vi "bar_code_reader.vi"() -> ()   [LabVIEW 2011]
doc: "This example shows how to use the IMAQ Read Barcode VI to read standard 1D barcodes.\n\nThe images are loaded with the Vision Acquisition Software Express VI."
uses:
  <vilib>/userDefined/High Color/IMAQdx.ctl
  <vilib>/vision/driver/IMAQdx.llb/IMAQdx Acquisition Mode.ctl
  <vilib>/vision/driver/IMAQdx.llb/IMAQdx Buffer Number Mode.ctl
  <vilib>/vision/NI_Vision_Development_Module.lvlib
  <vilib>/vision/driver/NI_Vision_Acquisition_Software.lvlib
panel:
  out "Code 4":string
  in  "Barcode Type":u32(ring)=6 items=["Reserved", "Codabar", "Code 39", "Code 93", "Code 128", "EAN 8", "EAN 13", "Interleaved 2 of 5", "MSI", "UPCA"]
  in  "Boolean 2":bool
  out "Code 3":string
  in  "Boolean":bool
  out "Code 2":string
  out "Acquisition Rate (frames/s)":dbl(knob) scale=0.0..110.0
  in  "stop 2":bool
  in  "Camera Name":T1
  out "Image":T2(plugin-control) caption="Draw a Rectangular Region of Interest on the BarCode"
  in  "Delay (ms)":i32(slide)=1446 max=3000 scale=0.0..100000.0
  # "This example requires Vision Acquisition Express VI to be installed"
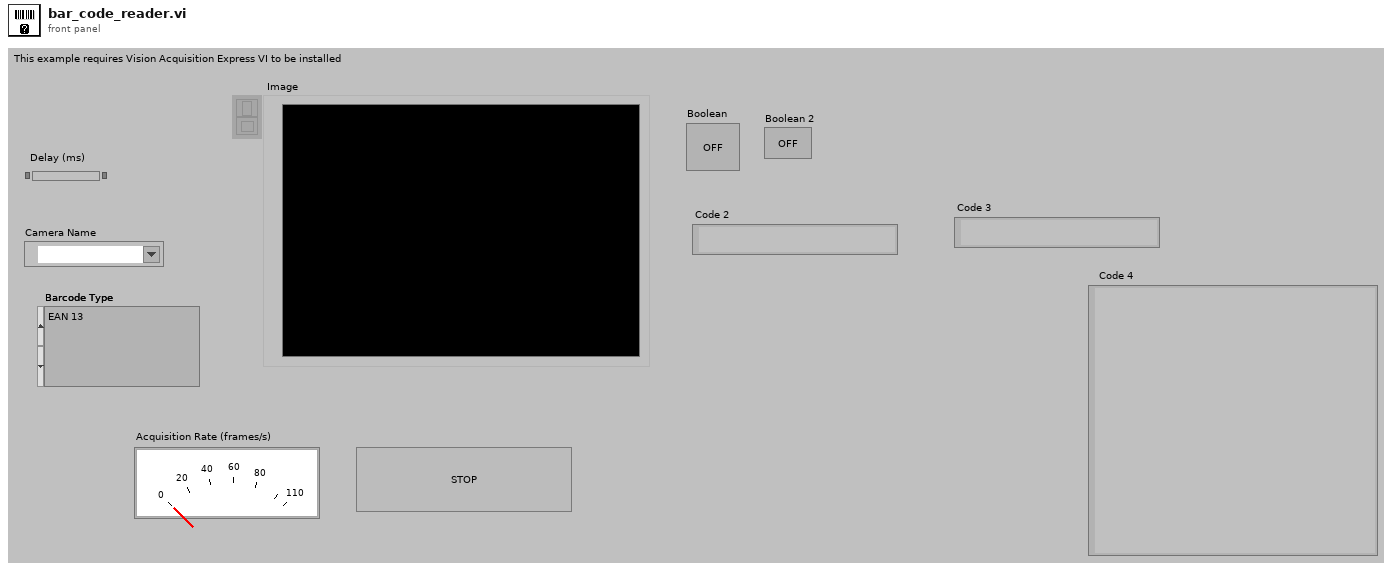
[diagram p1: front panel]
types:
  T1 = typedef "IMAQdx.ctl" = refnum<k21>
  T2 = typedef "IMAQ Image.ctl" = refnum<image>
  T3 = typedef "NI_Vision_Acquisition_Software.lvlib/IMAQdx Acquisition Mode.ctl" = enum32{"One Shot", "Continuous"}
  T4 = cluster{i32[], cluster{"Contour Type":u32, "ROI Type":u32, i32[]}[]}
  T5 = typedef "NI_Vision_Acquisition_Software.lvlib/IMAQdx Buffer Number Mode.ctl" = enum32{"Next", "Last", "Buffer Number"}
  T6 = cluster{"Special Char 1":string, "Special Char 2":string, "Confidence Level":sgl, "Barcode Type":u32}
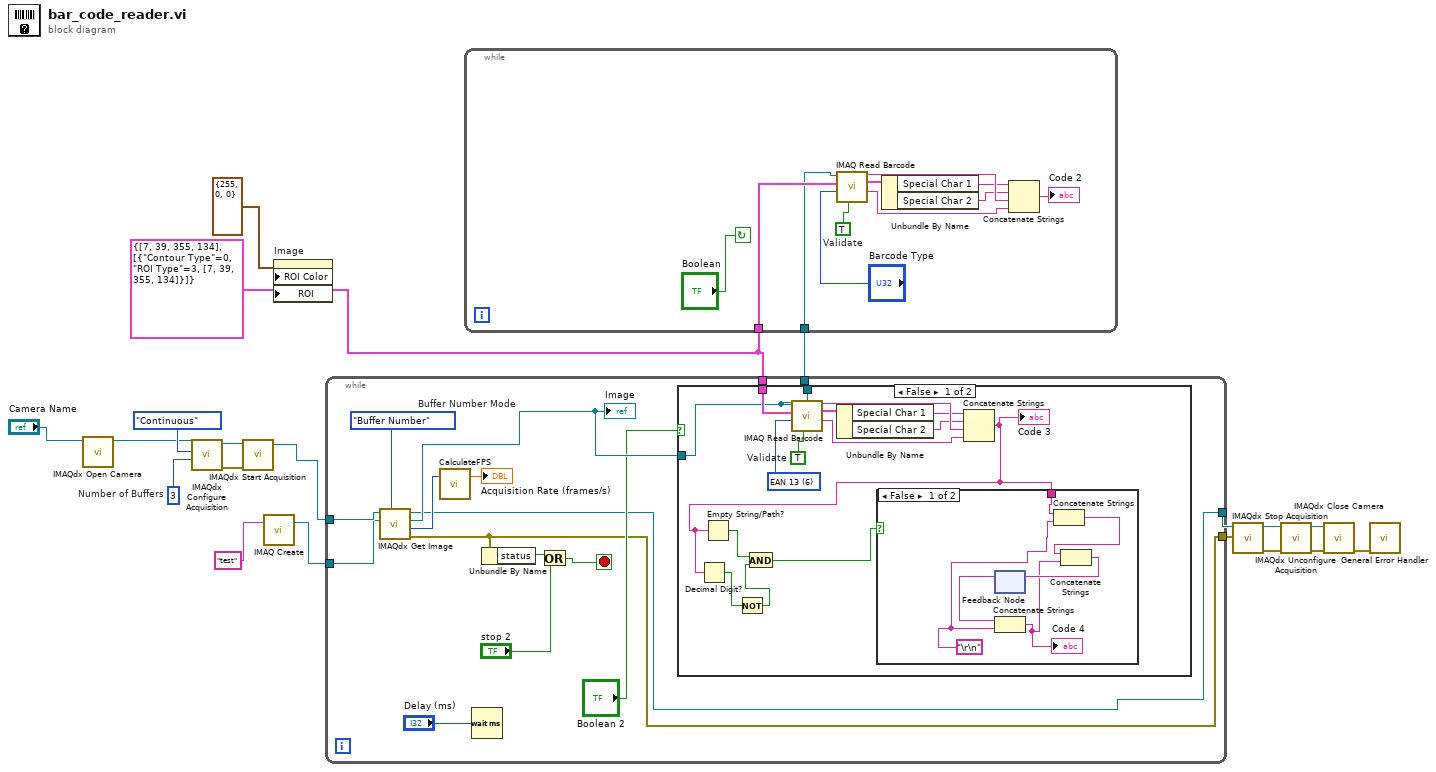
[diagram p0: block diagram]
diagram:
  w17 = u32 3  # Number of Buffers
  w1 = T4 {[7, 39, 355, 134], [{"Contour Type"=0, "ROI Type"=3, [7, 39, 355, 134]}]} ("ROI")
  n1 = call <vilib>:"IMAQdx Open Camera.vi"("Session In"="Camera Name") -> ("Session Out"=w13:T1)  [unwired: 2 in, 8 out]
  n2 = call <vilib>:"IMAQdx Configure Acquisition.vi"("Number of Buffers"=w17, "Continuous?"=IMAQdx_Acquisition_Mode."Continuous", "Session In"=w13) -> ("error out"=w15:errorcluster, "Session Out"=w14:T1)  [unwired: 1 in, 6 out]
  n3 = call <vilib>:"IMAQdx Start Acquisition.vi"("error in"=w15, "Session In"=w14) -> ("Session Out"=w4:T1)  [unwired: 9 out]
  n4 = call "IMAQ Create"("Image Name"="test") -> ("New Image"=w3:T2)  [unwired: 3 in, 2 out]
  n5 = property on="Image" class="ImageControl"("ROI Color"=cluster{"Red":u8, "Green":u8, "Blue":u8} {"Red"=255, "Green"=0, "Blue"=0}, "ROI"=w1) -> ()  [unwired: 2 in, 2 out]
  n6 = while {
    tunnel: [w21] -> w6
    tunnel: [w20] -> w5
    tunnel: w4 -> [w29]
    tunnel: w3 -> [w28]
    tunnel: [w24] -> w2
    tunnel: w1 -> [w23]
    stop <- w34 stop-if-true
    w32 = IMAQdx_Buffer_Number_Mode."Buffer Number"  # Buffer Number Mode
    n7 = call <vilib>:"IMAQdx Get Image.vi"("Buffer Number Mode (Next)"=w32, "Image In"=w28, "Session In"=w29) -> ("error out"=w20:errorcluster, "Buffer Number Out"=w30:u32, "Image Out"=w25:T2, "Session Out"=w21:T1)  [unwired: 2 in, 3 out]
    "Image" <- w25
    n8 = call "CalculateFPS.vi"("buffer number"=w30) -> ("acquired FPS"=→"Acquisition Rate (frames/s)":dbl)  [unwired: 2 out]
    n9 = Wait (ms)(milliseconds to wait="Delay (ms)") -> ()  [unwired: 1 out]
    n10 = Unbundle By Name(w20) -> ("status"=w33:bool)
    n11 = Or(x=w33, y="stop 2") -> (x .or. y?=w34:bool)
    n12 = case shown="False" "Boolean 2" {
      tunnel: w25 -> [w40 w55]
      tunnel: [w40 w55] -> w24
      tunnel: w23 -> [w41 _]
      frame False {
        w47 = TRUE  # Validate
        w42 = u32 6 items=["Reserved", "Codabar", "Code 39", "Code 93", "Code 128", "EAN 8", "EAN 13", "Interleaved 2 of 5", "MSI", "UPCA"] ("Barcode Type")
        n13 = call "IMAQ Read Barcode"("Validate"=w47, "Barcode Type"=w42, "ROI Descriptor"=w41, "Image"=w40) -> ("Checksum(s)"=w48:string, "Extra Info"=w43:T6, "String"=w46:string)  [unwired: 1 in, 4 out]
        n14 = Unbundle By Name(w43) -> ("Special Char 1"=w44:string, "Special Char 2"=w45:string)
        n15 = Concatenate Strings(w44, w45, w46, w48) -> (w39:string)
        "Code 3" <- w39
        n16 = Decimal Digit?(1:w39) -> (0:w36:bool)
        n17 = Empty String/Path?(string/path=w39) -> (empty?=w38:bool)
        n18 = Not(x=w36) -> (.not. x?=w35:bool)
        n19 = And(x=w38, y=w35) -> (x .and. y?=w37:bool)
        n20 = case shown="False" w37 {
          tunnel: w39 -> [w49 _]
          frame False {
            w51 = "\r\n"
            n21 = feedback #1() -> (w54:string)  [unwired: 1 in]
            n22 = Concatenate Strings(w54, w51) -> (w52:string)
            "Code 4" <- w52
            n23 = Concatenate Strings(w49, w51) -> (w50:string)
            n24 = Concatenate Strings(w50, w52) -> (w53:string)
            n25 = feedback-in #1(w53) -> ()
          }
          frame True {
          }
        }
      }
      frame True {
      }
    }
  }
  n26 = while {
    tunnel: w1 -> [w58]
    tunnel: w2 -> [w56]
    stop <- "Boolean" continue-if-true
    w65 = TRUE  # Validate
    n27 = call "IMAQ Read Barcode"("Validate"=w65, "Barcode Type"="Barcode Type", "ROI Descriptor"=w58, "Image"=w56) -> ("Checksum(s)"=w66:string, "Extra Info"=w60:T6, "String"=w63:string)  [unwired: 1 in, 4 out]
    n28 = Unbundle By Name(w60) -> ("Special Char 1"=w61:string, "Special Char 2"=w62:string)
    n29 = Concatenate Strings(w61, w62, w63, w66) -> (→"Code 2":string)
  }
  n30 = call <vilib>:"IMAQdx Stop Acquisition.vi"("error in"=w5, "Session In"=w6) -> ("error out"=w7:errorcluster, "Session Out"=w8:T1)  [unwired: 8 out]
  n31 = call <vilib>:"IMAQdx Unconfigure Acquisition.vi"("error in"=w7, "Session In"=w8) -> ("error out"=w10:errorcluster, "Session Out"=w9:T1)  [unwired: 8 out]
  n32 = call <vilib>:"IMAQdx Close Camera.vi"("error in"=w10, "Session In"=w9) -> ("error out"=w11:errorcluster)  [unwired: 9 out]
  n33 = call <vilib>:"General Error Handler.vi"("error in (no error)"=w11) -> ()  [unwired: 1 in, 14 out]
